vi "Sender.vi"() -> ()   [LabVIEW 2014]
uses:
  CommState.ctl
panel:
  in  "data in":dbl(slide) scale=0.0..10.0
  out "error out":errorcluster
  in  "stop":bool
  in  "IP Address":string="localhost"
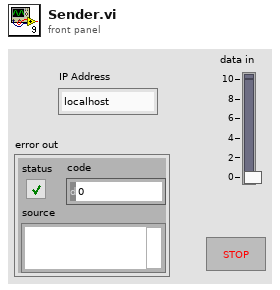
[diagram p1: front panel]
types:
  T1 = typedef "CommState.ctl" = enum16{"Disconnected", "Connected"}
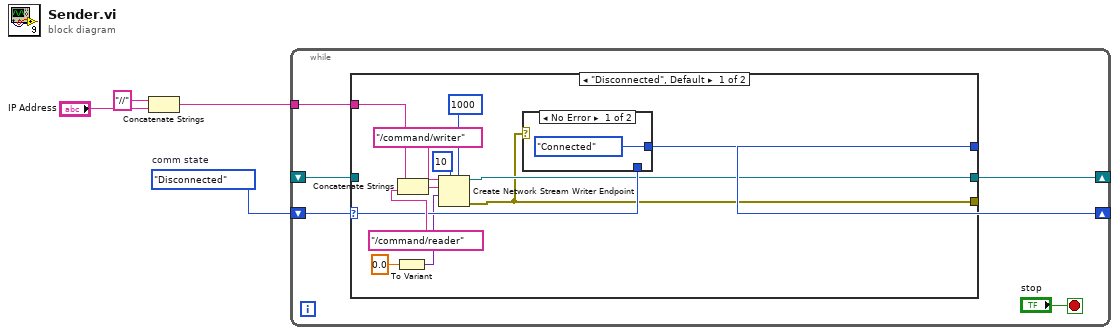
[diagram p0: block diagram]
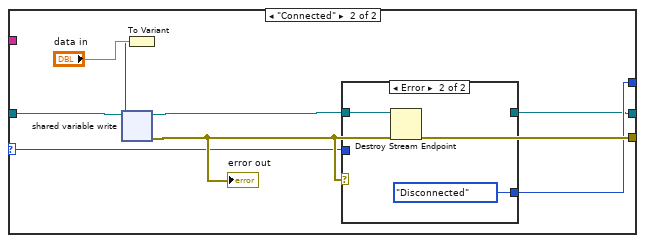
[diagram p3: hidden frame]
diagram:
  w4 = CommState."Disconnected"  # comm state
  n1 = Concatenate Strings("//" ("reader url"), "IP Address") -> (w1:string)
  n2 = while {
    tunnel: w1 -> [w9]
    shift-right: [w8] -> _
    shift-left: _ -> [w7]
    shift-right: [w5] -> _
    shift-left: w4 -> [w10]
    stop <- "stop" stop-if-true
    n3 = case shown="\"Disconnected\", Default" w10 {
      selector: w10 -> [w19 w29]
      tunnel: w9 -> [w22 _]
      tunnel: [w17 w27] -> w8
      tunnel: w7 -> [_ w32]
      tunnel: [w16 w31] -> _
      tunnel: [w20 w30] -> w5
      frame "Disconnected", Default {
        n4 = To Variant(anything=0.0) -> (Variant=w12:variant)
        n5 = Concatenate Strings(w22, "/command/reader" ("reader url")) -> (w15:string)
        n6 = Create Network Stream Writer Endpoint(5:1000 ("timeout in ms (-1)"), 7:10 ("reader buffer size"), 9:w12, 10:w15, 11:"/command/writer" ("writer name")) -> (0:w16:errorcluster, 3:w17:refnum<k21>)  [unwired: 2 in]
        n7 = case shown="No Error" w16 {
          tunnel: [CommState."Connected" ("comm state") w24] -> w20
          tunnel: w19 -> [_ w24]
          frame No Error {
          }
          frame Error {
          }
        }
      }
      frame "Connected" {
        n8 = To Variant(anything="data in") -> (Variant=w25:variant)
        n9 = shared-variable-write(w32, w25) -> (w28:refnum<k21>, w31:errorcluster)  [unwired: 2 in, 1 out]
        "error out" <- w31
        n10 = case shown="Error" w31 {
          tunnel: w29 -> [w34 _]
          tunnel: [w34 CommState."Disconnected" ("comm state")] -> w30
          tunnel: w28 -> [w33 w35]
          tunnel: [w33 _] -> w27
          frame No Error {
          }
          frame Error {
            n11 = Destroy Stream Endpoint(11:w35) -> ()  [unwired: 1 in, 1 out]
          }
        }
      }
    }
  }
